vi "union-intersection.vi"() -> ()   [LabVIEW 2011]
panel:
  in  "set_2":i32[](array[numeric])=[3, 4, 5, 6]
  in  "set_1":i32[](array[numeric])=[1, 2, 3]
  in  "Enum":enum16{"union", "intersection"}(ring)
  out "Output":i32[](array[numeric])
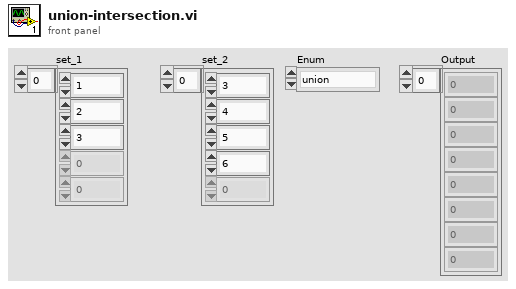
[diagram p1: front panel]
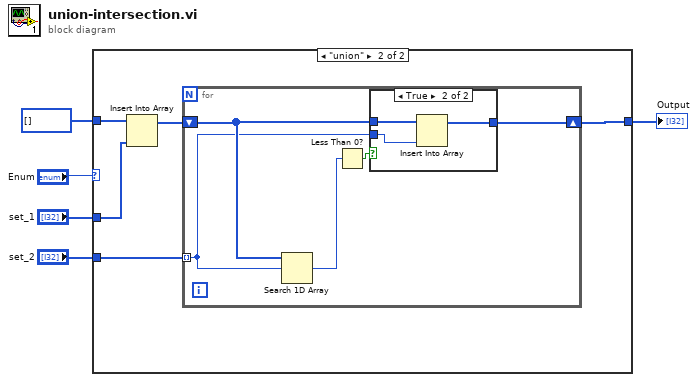
[diagram p0: block diagram]
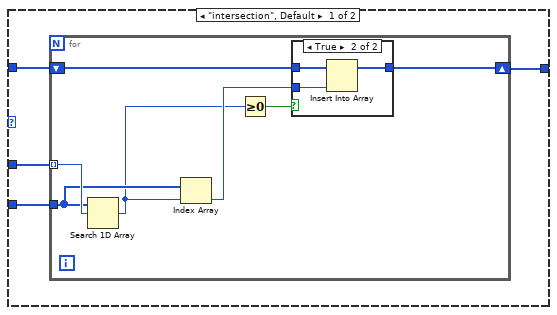
[diagram p2: hidden frame]
diagram:
  n1 = case shown="\"union\"" "Enum" {
    tunnel: "set_2" -> [w9 w23]
    tunnel: "set_1" -> [w8 w24]
    tunnel: i32[] [] -> [w7 w25]
    tunnel: [w6 w21] -> w2
    frame "intersection", Default {
      n2 = for {
        tunnel: w9 -> [w14]
        tunnel: w8 -> [w15] mode=indexing
        shift-right: [w13] -> w6
        shift-left: w7 -> [w16]
        n3 = Search 1D Array(1D array=w14, element=w15) -> (index of element=w10:i32)  [unwired: 1 in]
        n4 = Index Array(array=w14, index=w10) -> (element=w11:i32)
        n5 = Greater Or Equal To 0?(x=w10) -> (x >= 0?=w12:bool)
        n6 = case shown="True" w12 {
          tunnel: w16 -> [w17 w20]
          tunnel: w11 -> [_ w19]
          tunnel: [w17 w18] -> w13
          frame False {
          }
          frame True {
            n7 = Insert Into Array(array=w20, new element=w19) -> (w18:i32[])  [unwired: 1 in]
          }
        }
      }
    }
    frame "union" {
      n8 = Insert Into Array(array=w25, new element=w24) -> (w22:i32[])  [unwired: 1 in]
      n9 = for {
        tunnel: w23 -> [w26] mode=indexing
        shift-right: [w28] -> w21
        shift-left: w22 -> [w27]
        n10 = Search 1D Array(1D array=w27, element=w26) -> (index of element=w29:i32)  [unwired: 1 in]
        n11 = Less Than 0?(x=w29) -> (x < 0?=w30:bool)
        n12 = case shown="True" w30 {
          tunnel: w27 -> [w31 w34]
          tunnel: [w31 w33] -> w28
          tunnel: w26 -> [_ w32]
          frame False {
          }
          frame True {
            n13 = Insert Into Array(array=w34, new element=w32) -> (w33:i32[])  [unwired: 1 in]
          }
        }
      }
    }
  }
  "Output" <- w2
